vi "nRows.vi"(1 "array":i32[][](array[numeric])) -> (0 "Numeric":i32)   [LabVIEW 2013]
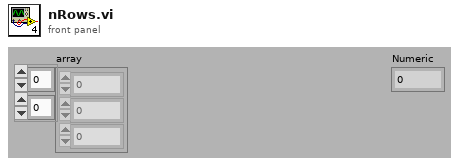
[diagram p1: front panel]
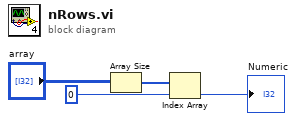
[diagram p0: block diagram]
diagram:
  n1 = Array Size(array="array") -> (size(s)=w1:i32[])
  n2 = Index Array(array=w1, index=0) -> (element=→"Numeric":i32)
